vi "get text before last open bracket.vi"(1 "Python String":string) -> (0 "Text After Last Open Bracket":string)   [LabVIEW 2020, in "jki_python_data_tools.lvlib"]
uses:
  jki_python_data_tools.lvlib
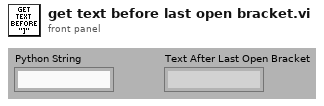
[diagram p1: front panel]
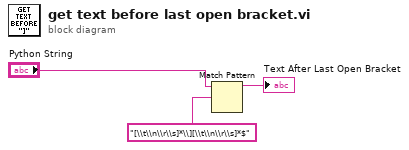
[diagram p0: block diagram]
diagram:
  n1 = Match Pattern(string="Python String", regular expression="[\\t\\n\\r\\s]*\\][\\t\\n\\r\\s]*$") -> (before substring=→"Text After Last Open Bracket":string)  [unwired: 1 in, 3 out]
